vi "controlLinearization.vi"(7 "Set":bool, 8 "error in":errorcluster, 9 "Enable":bool, 10 "axis in":u8, 11 "connection ID":refnum<k5>) -> (0 "error out":errorcluster, 1 "Enable out":bool, 2 "axis out":i32, 3 "connection ID":refnum<k5>)   [LabVIEW 2016, in "AMC_VIs.lvlib"]
doc: "Controls if linearization is enabled or not"
uses:
  AMC_VIs.lvlib
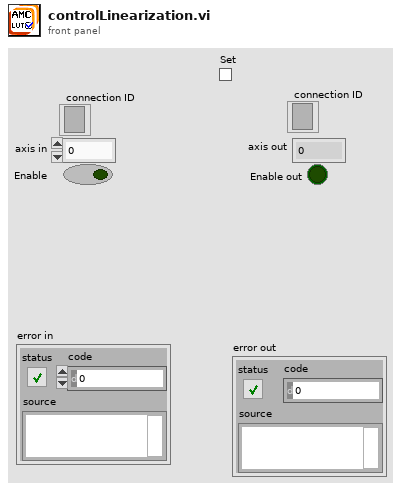
[diagram p1: front panel]
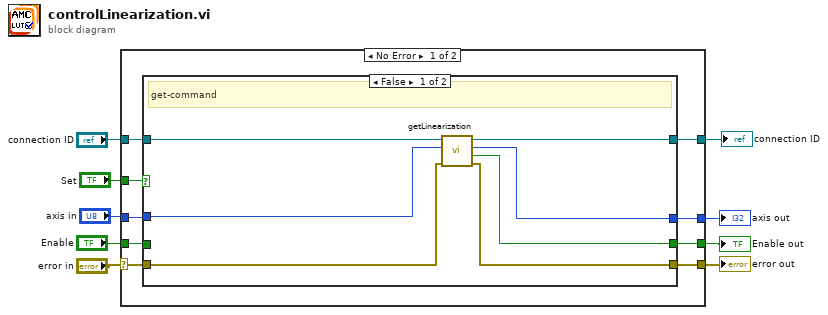
[diagram p0: block diagram]
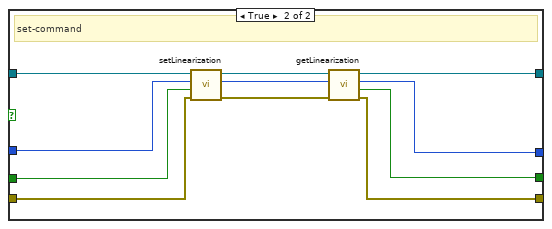
[diagram p2: hidden frame]
diagram:
  n1 = case shown="No Error" "error in" {
    selector: "error in" -> [w14 w40]
    tunnel: "axis in" -> [w18 w37]
    tunnel: [w11 w40] -> w8
    tunnel: "Enable" -> [w16 w38]
    tunnel: [w13 w38] -> w3
    tunnel: "Set" -> [w15 _]
    tunnel: [w12 w39] -> w6
    tunnel: "connection ID" -> [w17 w39]
    tunnel: [w10 w37] -> w1
    frame No Error {
      n2 = case shown="False" w15 {
        tunnel: w17 -> [w22 w36]
        tunnel: w18 -> [w21 w29]
        tunnel: w16 -> [_ w30]
        tunnel: w14 -> [w23 w33]
        tunnel: [w19 w26] -> w13
        tunnel: [w25 w34] -> w12
        tunnel: [w24 w31] -> w11
        tunnel: [w20 w27] -> w10
        frame False {
          # "get-command"
          n3 = call "getLinearization.vi"("error in"=w23, "axis"=w21, "connection ID"=w22) -> ("error out"=w24:errorcluster, "enabled"=w19:bool, "axis_out"=w20:i32, "connection ID"=w25:refnum<k5>)  [unwired: 5 in]
        }
        frame True {
          # "set-command"
          n4 = call "setLinearization.vi"("error in"=w33, "enable"=w30, "axis"=w29, "connection ID"=w36) -> ("error out"=w32:errorcluster, "axis_out"=w28:i32, "connection ID"=w35:refnum<k5>)  [unwired: 5 in]
          n5 = call "getLinearization.vi"("error in"=w32, "axis"=w28, "connection ID"=w35) -> ("error out"=w31:errorcluster, "enabled"=w26:bool, "axis_out"=w27:i32, "connection ID"=w34:refnum<k5>)  [unwired: 5 in]
        }
      }
    }
    frame Error {
    }
  }
  "error out" <- w8
  "axis out" <- w1
  "Enable out" <- w3
  "connection ID" <- w6
